vi "Create Frame Array.vi"(10 "Multi-Frame\nStructures":string[](array[string]), 11 "Refnum":refnum<vi>) -> (0 "Output References Array":refnum<vi>[](array[refnum]), 1 "Output Frame Array":T3(array[cluster]), 2 "Front Panel":T1, 3 "Block Diagram":T1, 4 "TopLevelDiagram":refnum<vi>, 5 "Documentation/Icon":T2, 6 "TLD UID":i32)   [LabVIEW 2024, in "VI Info.lvlib"]
doc: "This vi creates the Frame Array used for storing vi files in SVGs. Takes a path to a .vi file, returns the image data of the block diagram and front panel, an array of image info for each frame of multi-frame structures, an array of object refnums to each frame, and a cluster containing info on the vi icon and documentation."
uses:
  VI Info.lvlib
  <vilib>/picture/picture.llb/imagedata.ctl
  <vilib>/Utility/traverseref.llb/TRef TravTarget.ctl
  <vilib>/Utility/traverseref.llb/VI Scripting - Traverse.lvlib
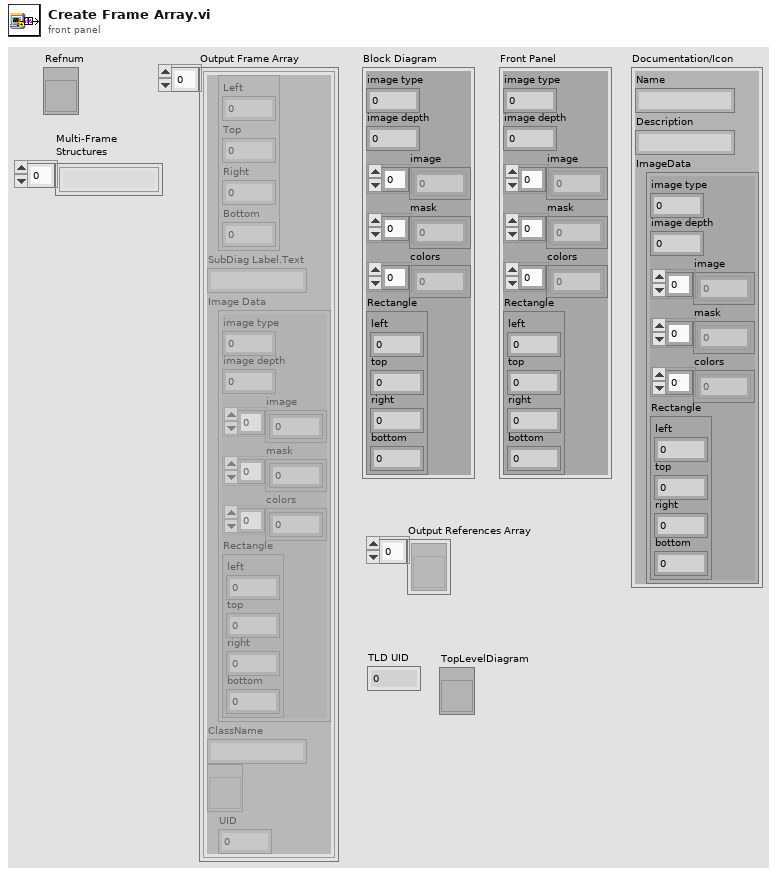
[diagram p1: front panel]
types:
  T1 = typedef "imagedata.ctl" = cluster{"image type":i32, "image depth":i32, "image":u8[], "mask":u8[], "colors":u32[], "Rectangle":cluster{"left":i16, "top":i16, "right":i16, "bottom":i16}}
  T2 = cluster{"Name":string, "Description":string, "ImageData":T1}
  T3 = cluster{cluster{"Left":i32, "Top":i32, "Right":u32, "Bottom":u32}, "SubDiag Label.Text":string, "Image Data":T1, "ClassName":string, refnum<vi>, "UID":i32}[]
  T4 = cluster{"Left":i32, "Top":i32, "Right":u32, "Bottom":u32}
  T5 = cluster{"left":i16, "top":i16, "right":i16, "bottom":i16}
  T6 = typedef "LVPositionTypeDef.ctl" = cluster{"Left":i32, "Top":i32}
  T7 = typedef "TRef TravTarget.ctl" = enum16{"FP", "BD", "Other"}
  T8 = typedef "LVBoundsTypeDef.ctl" = cluster{"Width":u32, "Height":u32}
  T9 = cluster{cluster{"Left":i32, "Top":i32, "Right":u32, "Bottom":u32}, "Frame Name":string, "Image Data":T1, "ClassName":string, refnum<vi>, "UID":i32}
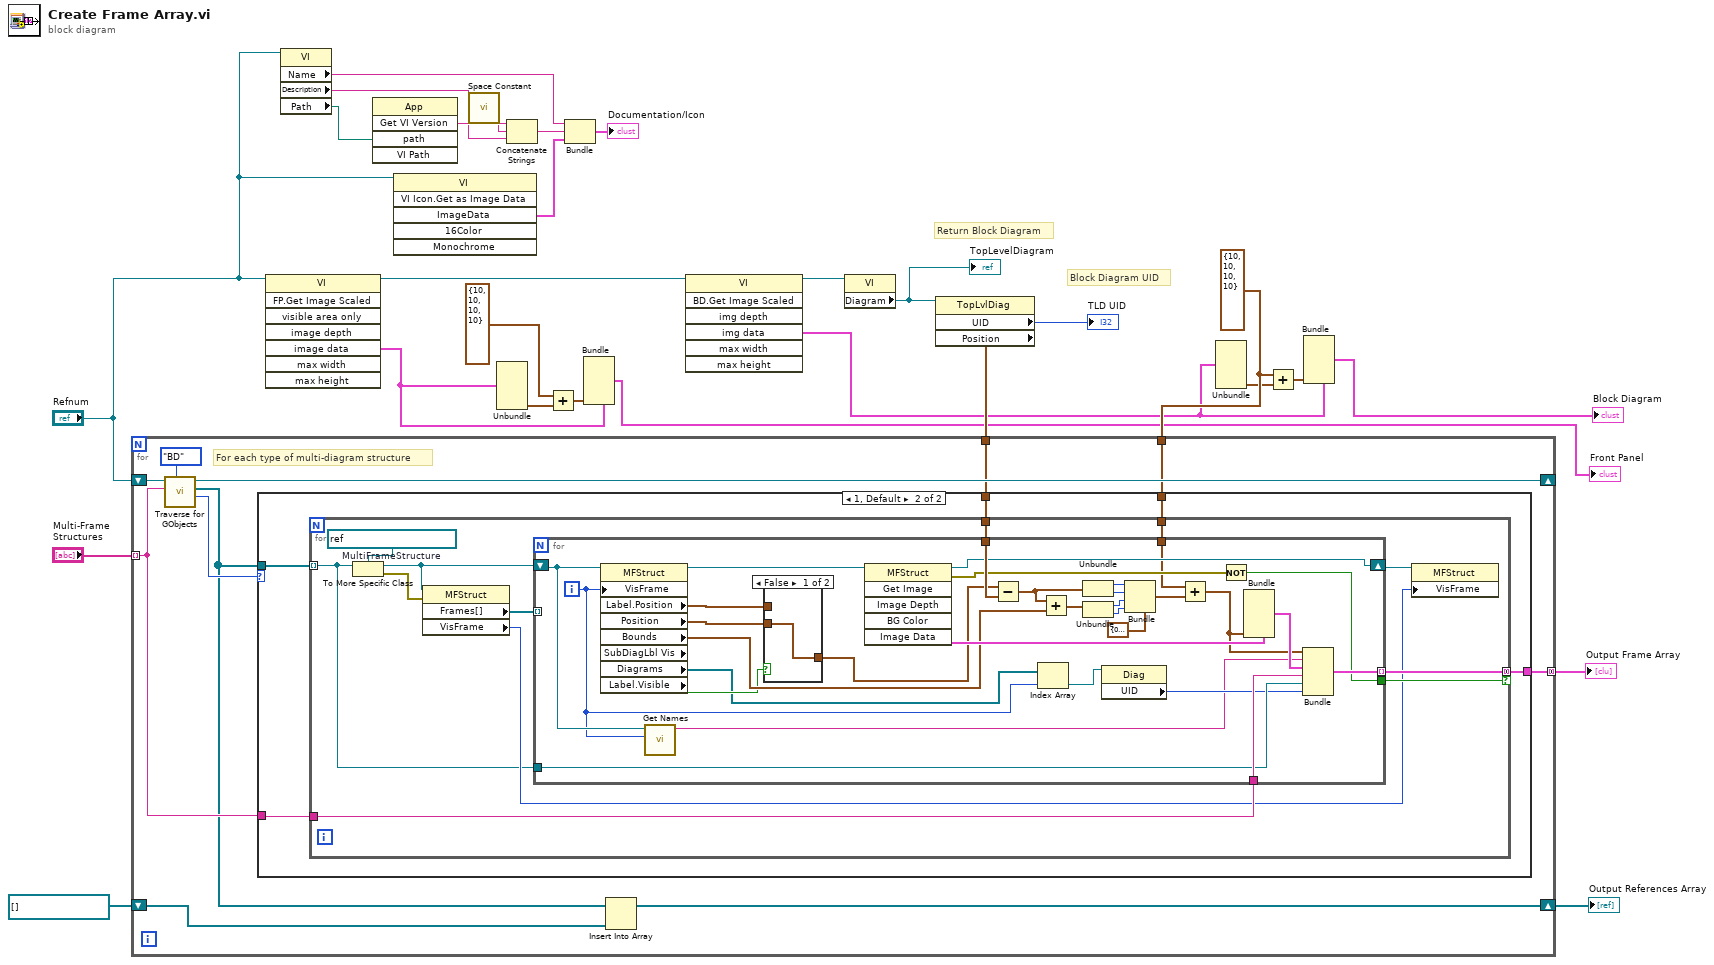
[diagram p0: block diagram]
diagram:
  w21 = T4 {"Left"=10, "Top"=10, "Right"=10, "Bottom"=10} ("output cluster")
  # "Block Diagram UID"
  # "Return Block Diagram"
  n1 = invoke class="VI" method="FP.Get Image Scaled"(reference="Refnum") -> (reference out=w16:refnum<vi>, "image data"=w20:T1)  [unwired: 7 in, 6 out]
  n2 = property class="VI"(reference="Refnum") -> ("Name"=w9:string, "Description"=w2:string, "Path"=w3:path)  [unwired: 1 in, 2 out]
  n3 = invoke class="App" method="Get VI Version"("path"=w3) -> ("GetVIVers"=w6:string)  [unwired: 4 in, 4 out]
  n4 = invoke class="VI" method="VI Icon.Get as Image Data"(reference="Refnum") -> ("ImageData"=w8:T1)  [unwired: 5 in, 5 out]
  n5 = call <vilib>:"Space Constant.vi"() -> ("String"=w1:string)
  n6 = Unbundle(w20) -> ("Rectangle"=w18:T5)  [unwired: 5 out]
  n7 = Concatenate Strings(w6, w1, w2) -> (w5:string)
  n8 = Add(x=T4 {"Left"=10, "Top"=10, "Right"=10, "Bottom"=10} ("output cluster"), y=w18) -> (x+y=w19:cluster{i32, i32, u32, u32})
  n9 = Bundle("Name"=w9, w5, "ImageData"=w8) -> (→"Documentation/Icon":cluster{"Name":string, string, "ImageData":T1})  [unwired: 1 in]
  n10 = Bundle(cluster=w20, "Rectangle"=w19) -> (→"Front Panel":T1)  [unwired: 5 in]
  n11 = invoke class="VI" method="BD.Get Image Scaled"(reference=w16) -> (reference out=w12:refnum<vi>, "img data"=w13:T1)  [unwired: 6 in, 5 out]
  n12 = property class="VI"(reference=w12) -> ("Diagram"=w27:refnum<vi>)  [unwired: 1 in, 2 out]
  "TopLevelDiagram" <- w27
  n13 = property class="TopLvlDiag"(reference=w27) -> ("UID"=→"TLD UID":i32, "Position"=w24:T6)  [unwired: 1 in, 2 out]
  n14 = for {
    tunnel: "Multi-Frame\nStructures" -> [w36] mode=indexing
    shift-right: [w37] -> _
    shift-left: "Refnum" -> [w39]
    tunnel: [w35] -> w22 mode=concatenating
    tunnel: w24 -> [w34]
    tunnel: w21 -> [w33]
    shift-right: [w30] -> w26
    shift-left: refnum<vi>[] [] ("References") -> [w31]
    # "For each type of multi-diagram structure"
    n15 = call <vilib>:"Traverse for GObjects.vi"("Traverse Target"=TRef_TravTarget."BD", "Class Name"=w36, "VI Refnum"=w39) -> ("# of Refs"=w32:i32, "References"=w29:refnum<vi>[], "dup VI Refnum"=w37:refnum<vi>)  [unwired: 5 in, 1 out]
    n16 = case shown="1, Default" w32 {
      tunnel: w29 -> [_ w44]
      tunnel: [_ w42] -> w35
      tunnel: w36 -> [_ w43]
      tunnel: w34 -> [_ w41]
      tunnel: w33 -> [_ w40]
      frame 0 {
      }
      frame 1, Default {
        n17 = for {
          tunnel: w44 -> [w45] mode=indexing
          tunnel: [w55] -> w42 mode=concatenating if=w54
          tunnel: w43 -> [w53]
          tunnel: w41 -> [w52]
          tunnel: w40 -> [w47]
          w56 = refnum<vi> refnum  # MultiFrameStructure
          n18 = To More Specific Class(target class=w56, reference=w45) -> (specific class reference=w51:refnum<vi>, error out=w50:errorcluster)  [unwired: 1 in]
          n19 = property class="MFStruct"(reference=w51, error in=w50) -> ("Frames[]"=w49:refnum<vi>[], "VisFrame"=w48:u32)  [unwired: 2 out]
          n20 = for {
            tunnel: [w82] -> w55 mode=indexing
            tunnel: [w81] -> w54
            tunnel: w53 -> [w79]
            tunnel: w52 -> [w78]
            tunnel: w49 -> [_] mode=indexing
            shift-right: [w69] -> w46
            shift-left: w51 -> [w59]
            tunnel: w47 -> [w66]
            tunnel: w45 -> [w63]
            i -> [w57]
            n21 = property class="MFStruct" props=["VisFrame", "Label", "Position", "Position", "Bounds", "SubDiagLbl Vis", "Diagrams", "Label", "Visible"](reference=w59, "VisFrame"=w57) -> (reference out=w74:refnum<vi>, "Label.Position"=w73:T6, "Position"=w72:T6, "Bounds"=w65:T8, "Diagrams"=w60:refnum<vi>[], "Label.Visible"=w64:bool)  [unwired: 1 in, 2 out]
            n22 = call "Get Names.vi"("Frame Index"=w57, "MFStruct Refnum"=w59) -> ("Frame Name"=w58:string)  [unwired: 9 in]
            n23 = case shown="False" w64 {
              tunnel: w73 -> [_ w89]
              tunnel: [w88 w89] -> w71
              tunnel: w72 -> [w88 _]
              frame False {
              }
              frame True {
              }
            }
            n24 = invoke class="MFStruct" method="Get Image"(reference=w74) -> (reference out=w69:refnum<vi>, error out=w70:errorcluster, "Image Data"=w76:T1)  [unwired: 5 in, 3 out]
            n25 = Subtract(x=w71, y=w78) -> (x-y=w77:T6)
            n26 = Index Array(array=w60, index=w57) -> (element=w62:refnum<vi>)
            n27 = Add(x=w77, y=w65) -> (x+y=w85:T8)
            n28 = Unbundle(w77) -> ("Left"=w86:i32, "Top"=w87:i32)
            n29 = Unbundle(w85) -> ("Width"=w84:u32, "Height"=w83:u32)
            n30 = property class="Diag"(reference=w62) -> ("UID"=w61:i32)  [unwired: 1 in, 2 out]
            n31 = Bundle(cluster=T4 {"Left"=0, "Top"=0, "Right"=0, "Bottom"=0}, "Left"=w86, "Top"=w87, "Right"=w84, "Bottom"=w83) -> (w68:T4)
            n32 = Add(x=w66, y=w68) -> (x+y=w67:T4)
            n33 = Not(x=w70) -> (.not. x?=w81:bool)
            n34 = Bundle(cluster=w76, "Rectangle"=w67) -> (w75:T1)  [unwired: 5 in]
            n35 = Bundle(w67, "Frame Name"=w58, "Image Data"=w75, "ClassName"=w79, w63, "UID"=w61) -> (w82:T9)  [unwired: 1 in]
          }
          n36 = property class="MFStruct"(reference=w46, "VisFrame"=w48) -> ()  [unwired: 1 in, 2 out]
        }
      }
    }
    n37 = Insert Into Array(array=w29, new element=w31) -> (w30:refnum<vi>[])  [unwired: 1 in]
  }
  "Output References Array" <- w26
  "Output Frame Array" <- w22
  n38 = Unbundle(w13) -> ("Rectangle"=w15:T5)  [unwired: 5 out]
  n39 = Add(x=w21, y=w15) -> (x+y=w14:cluster{i32, i32, u32, u32})
  n40 = Bundle(cluster=w13, "Rectangle"=w14) -> (→"Block Diagram":T1)  [unwired: 5 in]
